vi "After Each.vi"(8 "Error In":errorcluster, 11 "Reader In":refnum<class "Reader.lvclass">) -> (0 "Error Out":errorcluster)   [LabVIEW 2018, in "Tests.lvlib" / "Reader.lvlib"]
uses:
  Reader.lvlib
  src/LabPack/Public/Reader/Reader.lvclass
  src/LabPack/Public/Reader/Private/End by Value.vi
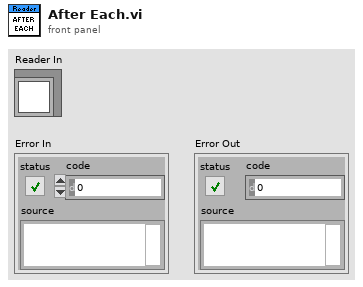
[diagram p1: front panel]
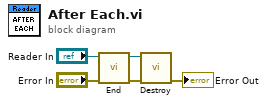
[diagram p0: block diagram]
diagram:
  n1 = call-poly "End.vi"("Error In"="Error In", "Reader In"="Reader In") -> ("Error Out"=w4:errorcluster, "Reader Out"=w5:refnum<class "Reader.lvclass">)  [unwired: 8 in]
  n2 = call "Destroy.vi"("Error In"=w4, "Reader"=w5) -> ("Error Out"=→"Error Out":errorcluster)  [unwired: 9 in]
